vi "RFH-fileextension_def.vi"(11 "Path in":path) -> (2 "File extention":string, 3 "Path with file extention":path)   [LabVIEW 2020, in "RFH-Reflection_File_Handler.lvlib"]
uses:
  RFH-Reflection_File_Handler.lvlib
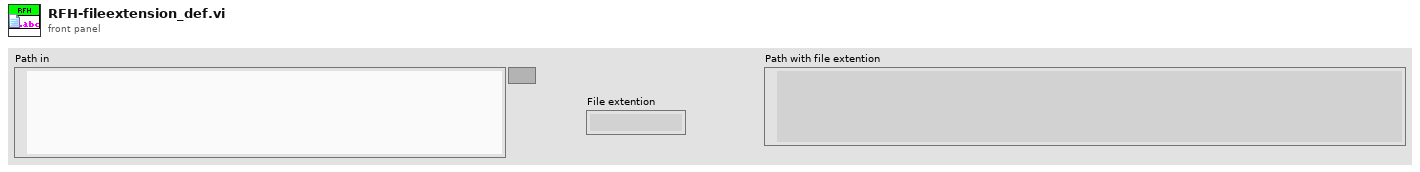
[diagram p1: front panel]
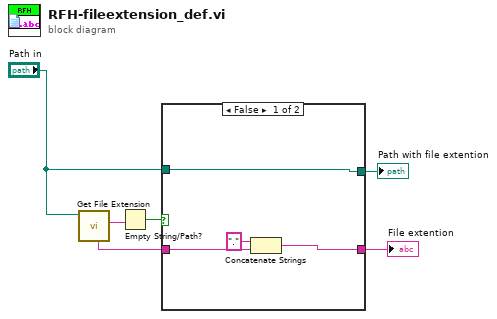
[diagram p0: block diagram]
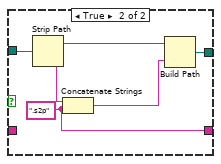
[diagram p2: hidden frame]
diagram:
  n1 = call <vilib>:"Get File Extension.vi"("file"="Path in") -> ("lowercase file extension"=w4:string, "unmodified file extension"=w1:string)  [unwired: 6 in, 3 out]
  n2 = Empty String/Path?(string/path=w4) -> (empty?=w3:bool)
  n3 = case shown="False" w3 {
    tunnel: [w10 w15] -> w6
    tunnel: [w8 w14] -> w5
    tunnel: "Path in" -> [w10 w13]
    tunnel: w1 -> [w9 _]
    frame False {
      n4 = Concatenate Strings("." ("string"), w9) -> (w8:string)
    }
    frame True {
      w14 = ".s2p"
      n5 = Strip Path(path=w13) -> (stripped path=w12:path, name=w11:string)
      n6 = Concatenate Strings(w11, w14) -> (w16:string)
      n7 = Build Path(base path=w12, name or relative path=w16) -> (appended path=w15:path)
    }
  }
  "Path with file extention" <- w6
  "File extention" <- w5
